vi "Run Profiled Cascade.vi"(8 "Cascade Start Position":dbl, 9 "Iteration":i32, 10 "Velocity Profile":dbl[](array[numeric]), 11 "Cascade In":T1={"DeviceStatus"={"status"=FALSE, "code"=0, "source"=""}, "Type"=enum."PWM", "PWM"={"PWM Channel"=enum."Invalid", "DeadBand"={"Name"="", "maxPositivePwm"=0, "minPositivePwm"=0, "centerPwm"=0, "maxNegativePwm"=0, "minNegativePwm"=0, "angularRange"=0}}, "CAN"={"Device Number"=0, "SetOutput VI Ref"=variant(refnum<vi> refnum), "GetOutput VI Ref"=variant(refnum<vi> refnum), "Enable VI Ref"=variant(refnum<vi> refnum), "Disable VI Ref"=variant(refnum<vi> refnum), "Data"=variant}, "Invert"=FALSE, "DIO PWM"={"PWM \"Enable\" Channel"=enum."Invalid", "DIOChannel"=enum."Invalid", "PWM Rate"=0.0}}) -> (3 "Cascade Out":T1={"DeviceStatus"={"status"=FALSE, "code"=0, "source"=""}, "Type"=enum."PWM", "PWM"={"PWM Channel"=enum."Invalid", "DeadBand"={"Name"="", "maxPositivePwm"=0, "minPositivePwm"=0, "centerPwm"=0, "maxNegativePwm"=0, "minNegativePwm"=0, "angularRange"=0}}, "CAN"={"Device Number"=0, "SetOutput VI Ref"=variant(refnum<vi> refnum), "GetOutput VI Ref"=variant(refnum<vi> refnum), "Enable VI Ref"=variant(refnum<vi> refnum), "Disable VI Ref"=variant(refnum<vi> refnum), "Data"=variant}, "Invert"=FALSE, "DIO PWM"={"PWM \"Enable\" Channel"=enum."Invalid", "DIOChannel"=enum."Invalid", "PWM Rate"=0.0}})   [LabVIEW 2020]
uses:
  <vilib>/Rock Robotics/WPI/MotorControl/WPI_MotorControlDeviceRef.ctl
  <vilib>/Rock Robotics/WPI/MotorControl/WPI_MotorControlType.ctl
  <vilib>/Rock Robotics/SystemInterfaces/DIO/FPGA_DIOPWMChannel.ctl
  <vilib>/Rock Robotics/WPI/PWM/WPI_PWMDeadband.ctl
  <vilib>/Rock Robotics/SystemInterfaces/DIO/FPGA_DIOChannel.ctl
  <vilib>/Rock Robotics/WPI/ThirdParty/REV Robotics/REVLib/Typedef/Spark MAX Control Type.ctl
panel:
  out "Velocity":cluster{dbl, dbl, "Arbitrary Feedforward":dbl}(graph)
  out "Position":cluster{dbl, "Sensor Position":dbl}(graph)
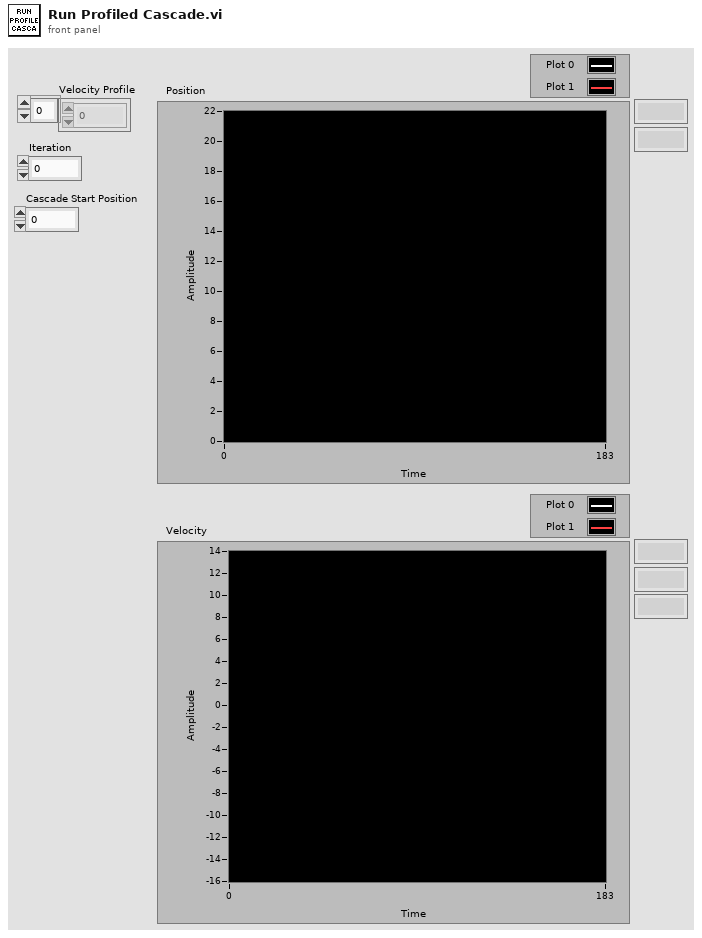
[diagram p1: front panel]
types:
  T1 = typedef "WPI_MotorControlDeviceRef.ctl" = cluster{"DeviceStatus":errorcluster, "Type":T2, "PWM":cluster{"PWM Channel":T3, "DeadBand":T4}, "CAN":cluster{"Device Number":u8, "SetOutput VI Ref":variant, "GetOutput VI Ref":variant, "Enable VI Ref":variant, "Disable VI Ref":variant, "Data":variant}, "Invert":bool, "DIO PWM":cluster{"PWM \"Enable\" Channel":T3, "DIOChannel":T5, "PWM Rate":dbl}}
  T2 = typedef "WPI_MotorControlType.ctl" = enum16{"PWM", "CAN", "DIO PWM"}
  T3 = typedef "FPGA_DIOPWMChannel.ctl" = enum8{"PWM 0", "PWM 1", "PWM 2", "PWM 3", "PWM 4", "PWM 5", "PWM 6", "PWM 7", "PWM 8", "PWM 9", "PWM MXP 0", "PWM MXP 1", "PWM MXP 2", "PWM MXP 3", "PWM MXP 4", "PWM MXP 5", "PWM MXP 6", "PWM MXP 7", "PWM MXP 8", "PWM MXP 9", "Invalid"}
  T4 = typedef "WPI_PWMDeadband.ctl" = cluster{"Name":string, "maxPositivePwm":i32, "minPositivePwm":i32, "centerPwm":i32, "maxNegativePwm":i32, "minNegativePwm":i32, "angularRange":u16}
  T5 = typedef "FPGA_DIOChannel.ctl" = enum8{"DIO 0", "DIO 1", "DIO 2", "DIO 3", "DIO 4", "DIO 5", "DIO 6", "DIO 7", "DIO 8", "DIO 9", "DIO MXP 0", "DIO MXP 1", "DIO MXP 2", "DIO MXP 3", "DIO MXP 4", "DIO MXP 5", "DIO MXP 6", "DIO MXP 7", "DIO MXP 8", "DIO MXP 9", "DIO MXP 10", "DIO MXP 11", "DIO MXP 12", "DIO MXP 13", "DIO MXP 14", "DIO MXP 15", "SPI Port CS1", "SPI Port CS2", "SPI Port CS3", "SPI Port MISO", "SPI Port MOSI", "Invalid"}
  T6 = typedef "Spark MAX Control Type.ctl" = enum16{"Percent VBus", "Voltage", "Velocity", "Position", "Smart Motion", "Current", "Smart Velocity"}
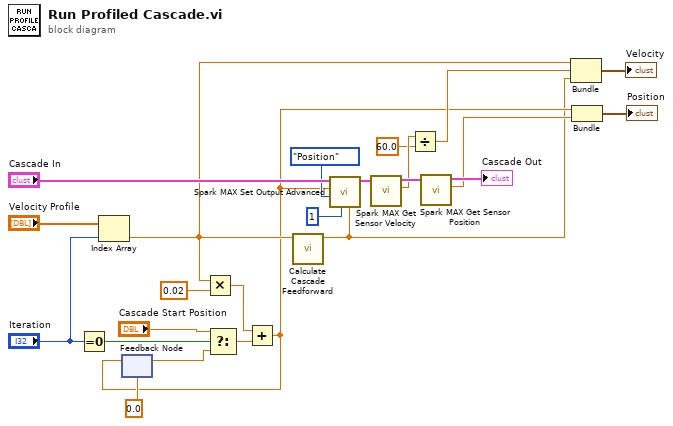
[diagram p0: block diagram]
diagram:
  n1 = Equal To 0?(x="Iteration") -> (x = 0?=w19:bool)
  n2 = Index Array(array="Velocity Profile", index="Iteration") -> (element=w10:dbl)
  n3 = feedback #1(0.0 ("t")) -> (w14:dbl)
  n4 = Multiply(x=w10, y=0.02) -> (x*y=w17:dbl)
  n5 = Select(t="Cascade Start Position", s=w19, f=w14) -> (s? t:f=w15:dbl)
  n6 = Add(x=w17, y=w15) -> (x+y=w3:dbl)
  n7 = feedback-in #1(w3) -> ()
  n8 = call "Calculate Cascade Feedforward.vi"("Setpoint"=w10) -> ("Arbitrary Feedforward"=w1:dbl)  [unwired: 10 in]
  n9 = call <vilib>:"Spark MAX Set Output Advanced.vi"("Arbitrary Feed Forward (0)"=w1, "PIDF Slot (0)"=1, "Control Mode"=Spark_MAX_Control_Type."Position", "Setpoint"=w3, "MotorControlDevRef"="Cascade In") -> ("MotorControlDevRef"=w9:T1)  [unwired: 5 in, 1 out]
  n10 = call <vilib>:"Spark MAX Get Sensor Velocity.vi"("MotorControlDevRef in"=w9) -> ("Sensor Velocity"=w6:dbl, "MotorControlDevRef out"=w8:T1)  [unwired: 7 in, 2 out]
  n11 = Divide(x=w6, y=60.0) -> (x/y=w4:dbl)
  n12 = call <vilib>:"Spark MAX Get Sensor Position.vi"("MotorControlDevRef in"=w8) -> ("Sensor Position"=w12:dbl, "MotorControlDevRef out"=→"Cascade Out":T1)  [unwired: 7 in, 2 out]
  n13 = Bundle(w10, w4, "Arbitrary Feedforward"=w1) -> (→"Velocity":cluster{dbl, dbl, "Arbitrary Feedforward":dbl})  [unwired: 1 in]
  n14 = Bundle(w3, "Sensor Position"=w12) -> (→"Position":cluster{dbl, "Sensor Position":dbl})  [unwired: 1 in]
